vi "MFLI_api -- V2.vi"(4 "Oscillator (0)":u16, 5 "MFLI Address":string="DEV3523", 6 "delay-circle(msec)":i64, 7 "MFLI frontend action":T1, 8 "Error In":errorcluster, 10 "Freq IN (Hz)":dbl=40000.0 format="%#_13g", 11 "Handle In":T2 {"Handle" format="0x%08x"; "Conn" format="0x%08x"}) -> (0 "Error Out":errorcluster, 1 "z out (V)":cdb, 2 "Freq out (Hz)":dbl=40000.0 format="%#_13g", 3 "Handle Out":T2 {"Handle" format="0x%08x"; "Conn" format="0x%08x"})   [LabVIEW 2018]
uses:
  Applications/National Instruments/LabVIEW 2019 64-bit/instr.lib/Zurich Instruments LabOne/Zurich Instruments LabOne.lvlib
  MFLI frontend action.ctl
  Applications/National Instruments/LabVIEW 2019 64-bit/instr.lib/Zurich Instruments LabOne/Public/ziTypeHandle.ctl
panel:
  out "Selected Device":string="DEV3523"
  in  "timeconstant (s)":dbl=0.006
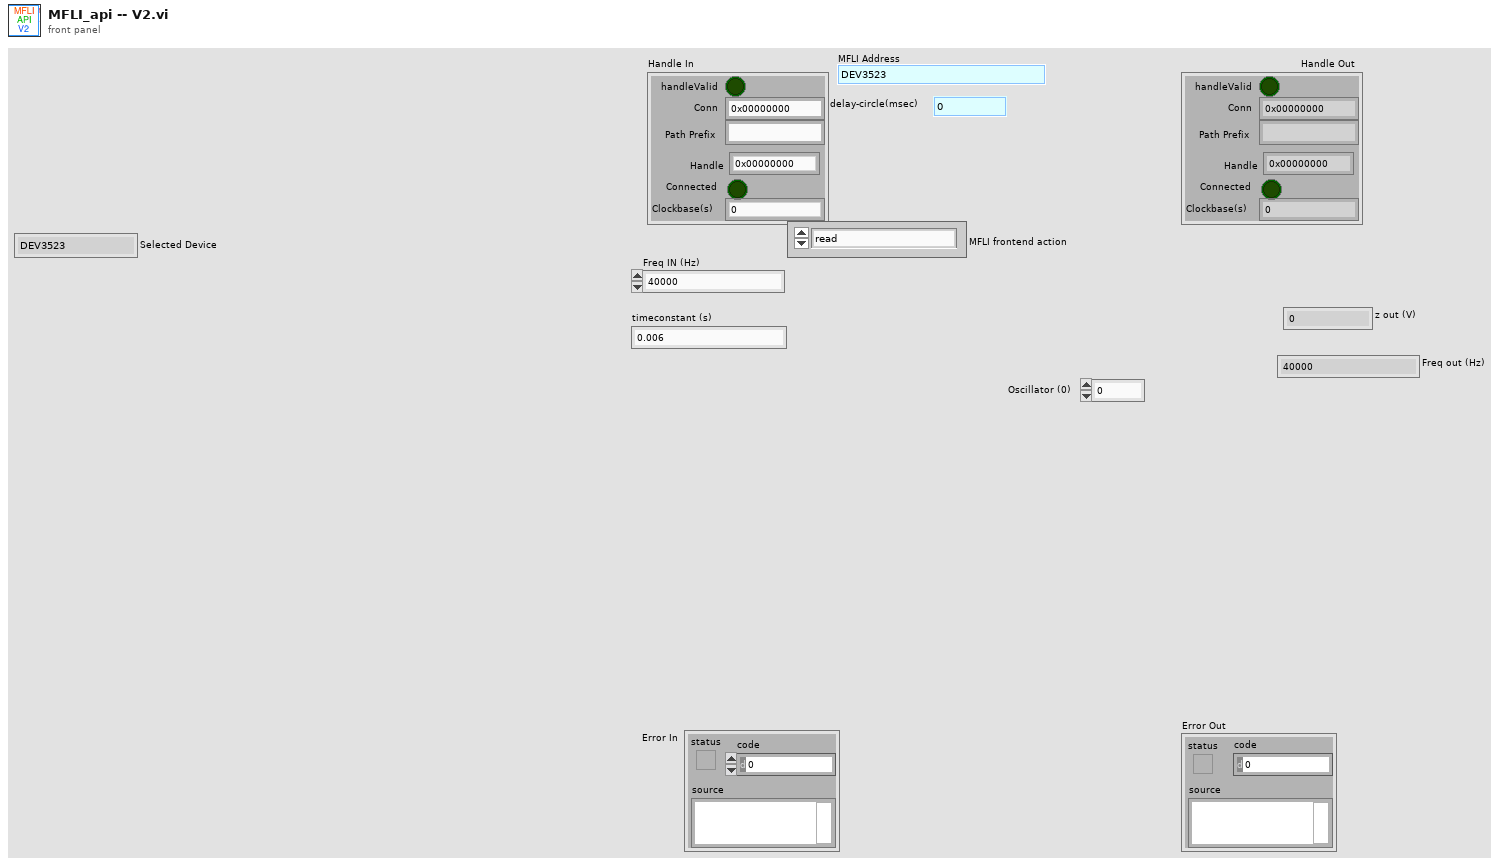
[diagram p1: front panel]
types:
  T1 = typedef "MFLI frontend action.ctl" = enum16{"read", "writeread", "open", "close", "write"}
  T2 = typedef "Zurich Instruments LabOne.lvlib/ziTypeHandle.ctl" = cluster{"handleValid":bool, "Conn":u64, "Path Prefix":string, "Handle":u64, "Connected":bool, "Clockbase(s)":dbl}
  T3 = typedef "Zurich Instruments LabOne.lvlib/ziTypeDemodSampleSingle.ctl" = cluster{"Timestamps (ticks)":u64, "X (Vrms)":dbl, "Y (Vrms)":dbl, "Osc Phase (deg)":dbl, "Freq (Hz)":dbl, "DIO":u32, "AuxIn0 (V)":dbl, "AuxIn1 (V)":dbl, "Trigger":u32}
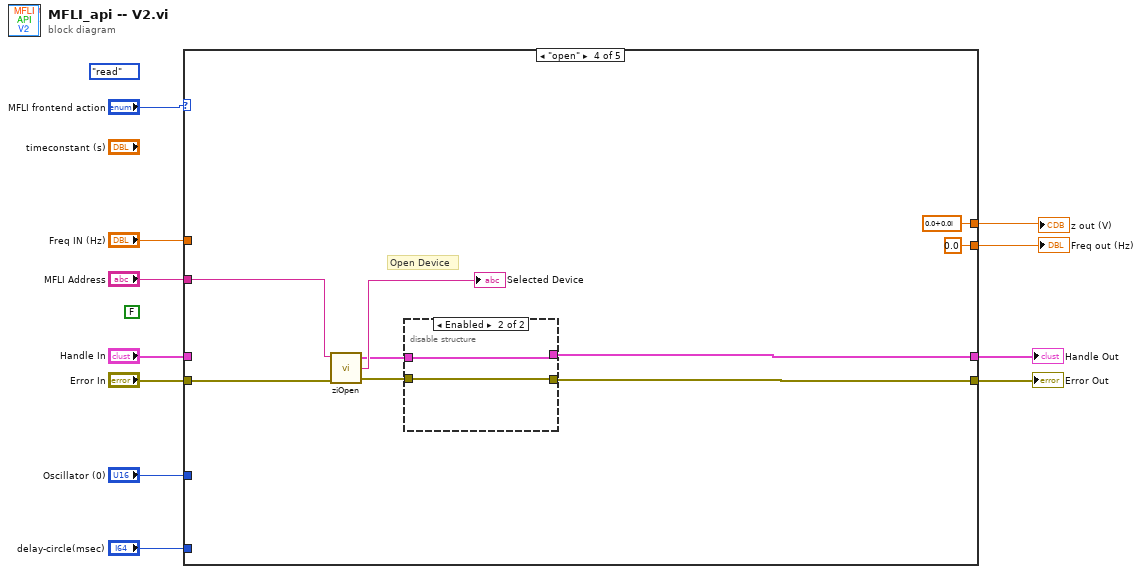
[diagram p0: block diagram]
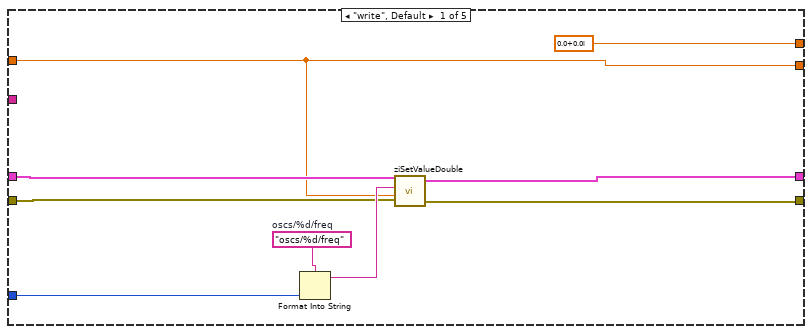
[diagram p2: hidden frame]
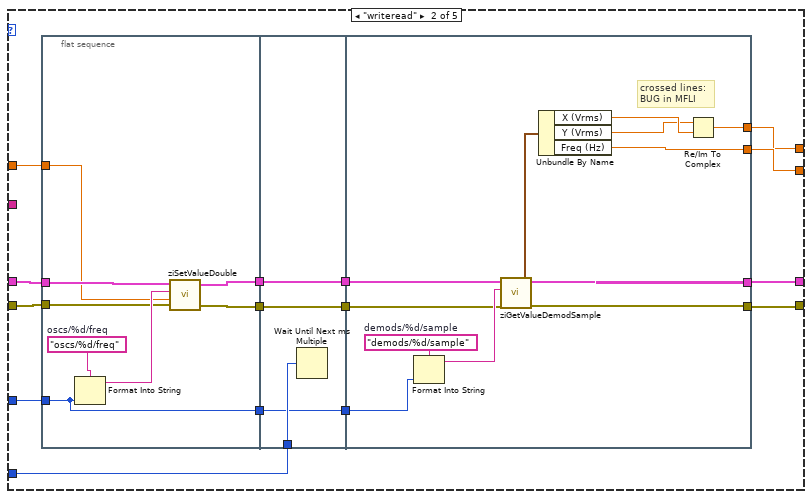
[diagram p3: hidden frame]
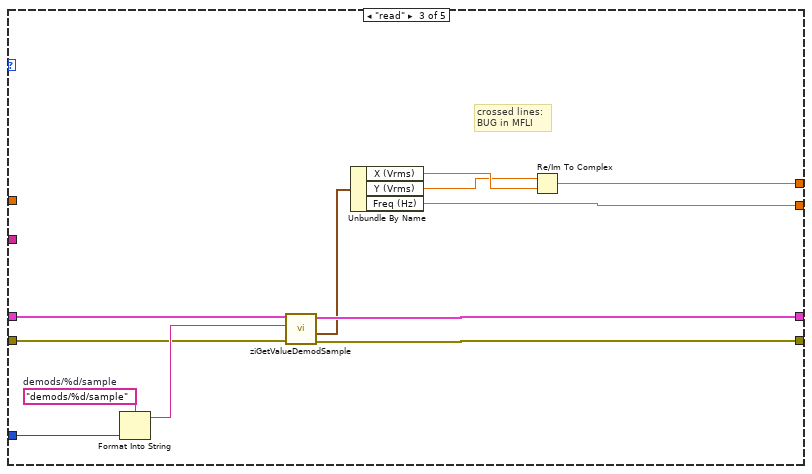
[diagram p4: hidden frame]
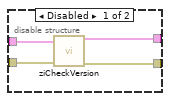
[diagram p5: hidden frame]
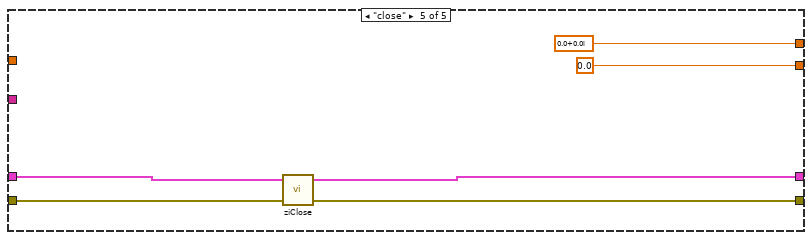
[diagram p6: hidden frame]
diagram:
  (unwired) MFLI_frontend_action."read" ("MFLI frontend action")
  (unwired) FALSE
  n1 = case shown="\"open\"" "MFLI frontend action" {
    tunnel: [w16 w33 w71 w75 w89] -> w11
    tunnel: [w15 w32 w70 w74 w90] -> w10
    tunnel: [cdb 0.0+0.0i w23 w64 cdb 0.0+0.0i cdb 0.0+0.0i] -> w9
    tunnel: "Handle In" -> [w18 w35 w63 _ w92]
    tunnel: "Error In" -> [w17 w34 w62 w77 w91]
    tunnel: "Oscillator (0)" -> [w14 w30 w61 _ _]
    tunnel: [w13 w24 w60 0.0 ("Freq (Hz)") 0.0 ("Freq (Hz)")] -> w5
    tunnel: "MFLI Address" -> [_ _ _ w76 _]
    tunnel: "Freq IN (Hz)" -> [w13 w31 _ _ _]
    tunnel: "delay-circle(msec)" -> [_ w25 _ _ _]
    frame "write", Default {
      w20 = "oscs/%d/freq"  # oscs/%d/freq
      n2 = Format Into String(format string=w20, w14) -> (resulting string=w19:string)  [unwired: 2 in, 1 out]
      n3 = call "ziSetValueDouble.vi"("Error In"=w17, "Value"=w13, "Path"=w19, "Handle In"=w18) -> ("Error Out"=w15:errorcluster, "Handle Out"=w16:T2)  [unwired: 1 in]
    }
    frame "writeread" {
      n4 = flat-sequence {
        tunnel: w35 -> [w41]
        tunnel: w34 -> [w40]
        tunnel: w31 -> [w37]
        tunnel: w30 -> [w36]
        tunnel: [w39] -> w29
        tunnel: [w38] -> w28
        tunnel: [w36] -> w22
        tunnel: w29 -> [w47]
        tunnel: w28 -> [w46]
        tunnel: [w47] -> w27
        tunnel: [w46] -> w26
        tunnel: w25 -> [w45]
        tunnel: w22 -> [w44]
        tunnel: [w44] -> w21
        tunnel: [w51] -> w32
        tunnel: [w49] -> w33
        tunnel: w27 -> [w50]
        tunnel: w26 -> [w52]
        tunnel: [w54] -> w24
        tunnel: [w53] -> w23
        tunnel: w21 -> [w48]
        frame #0 {
          w43 = "oscs/%d/freq"  # oscs/%d/freq
          n5 = Format Into String(format string=w43, w36) -> (resulting string=w42:string)  [unwired: 2 in, 1 out]
          n6 = call "ziSetValueDouble.vi"("Error In"=w40, "Value"=w37, "Path"=w42, "Handle In"=w41) -> ("Error Out"=w38:errorcluster, "Handle Out"=w39:T2)  [unwired: 1 in]
        }
        frame #1 {
          n7 = Wait Until Next ms Multiple(millisecond multiple=w45) -> ()  [unwired: 1 out]
        }
        frame #2 {
          w58 = "demods/%d/sample"  # demods/%d/sample
          # "crossed lines:\nBUG in MFLI"
          n8 = Format Into String(format string=w58, w48) -> (resulting string=w59:string)  [unwired: 2 in, 1 out]
          n9 = call "ziGetValueDemodSample.vi"("error in"=w52, "Path"=w59, "Handle In"=w50) -> ("error out"=w51:errorcluster, "Demod Sample Out"=w57:T3, "Handle Out"=w49:T2)  [unwired: 2 in]
          n10 = Unbundle By Name(w57) -> ("X (Vrms)"=w56:dbl, "Y (Vrms)"=w55:dbl, "Freq (Hz)"=w54:dbl)
          n11 = Re/Im To Complex(1:w56, 2:w55) -> (0:w53:cdb)
        }
      }
    }
    frame "read" {
      w68 = "demods/%d/sample"  # demods/%d/sample
      # "crossed lines:\nBUG in MFLI"
      n12 = Format Into String(format string=w68, w61) -> (resulting string=w69:string)  [unwired: 2 in, 1 out]
      n13 = call "ziGetValueDemodSample.vi"("error in"=w62, "Path"=w69, "Handle In"=w63) -> ("error out"=w70:errorcluster, "Demod Sample Out"=w67:T3, "Handle Out"=w71:T2)  [unwired: 2 in]
      n14 = Unbundle By Name(w67) -> ("X (Vrms)"=w66:dbl, "Y (Vrms)"=w65:dbl, "Freq (Hz)"=w60:dbl)
      n15 = Re/Im To Complex(1:w66, 2:w65) -> (0:w64:cdb)
    }
    frame "open" {
      # "Open Device"
      n16 = call "ziOpen.vi"("Error In"=w77, "Address"=w76) -> ("Error Out"=w80:errorcluster, "Selected Device"=→"Selected Device":string, "HandleOut"=w78:T2)  [unwired: 2 in]
      n17 = disable-structure shown="Enabled" {
        disable-tunnel: w80 -> [w84 w85]
        disable-tunnel: [w83 w85] -> w74
        disable-tunnel: [w82 w86] -> w75
        disable-tunnel: w78 -> [w81 w86]
        frame Disabled {
          n18 = call "ziCheckVersion.vi"("Handle In"=w81, "Error In"=w84) -> ("Handle Out"=w82:T2, "Error Out"=w83:errorcluster)  [unwired: 11 in, 1 out]
        }
        frame Enabled {
        }
      }
    }
    frame "close" {
      n19 = call "ziClose.vi"("Error In"=w91, "Handle In"=w92) -> ("Error Out"=w90:errorcluster, "Handle Out"=w89:T2)  [unwired: 2 in]
    }
  }
  "Handle Out" <- w11
  "Error Out" <- w10
  "z out (V)" <- w9
  "Freq out (Hz)" <- w5
